vi "Elevator Controller.vi"(8 "error in (no error)":errorcluster, 11 "View Model":T1) -> (0 "error out":errorcluster)   [LabVIEW 2017]
doc: "Handles all elevator operations."
uses:
  View Model/Controls/View Model.ctl
  Configuration/Controls/Config Model.ctl
  Configuration/Controls/Config Data.ctl
  Error Handler/Controls/Error Model.ctl
  Error Handler/Controls/Error Data.ctl
  Error Handler/Controls/Error Type.ctl
  View Model/Controls/Shared Model.ctl
  Controls/Elevator Model.ctl
  Controls/Elevator Location.ctl
  Controls/Elevator CMD Data.ctl
  Controls/Elevator Commands.ctl
  Controls/Elevator Overhead.ctl
  Controls/Elevator States.ctl
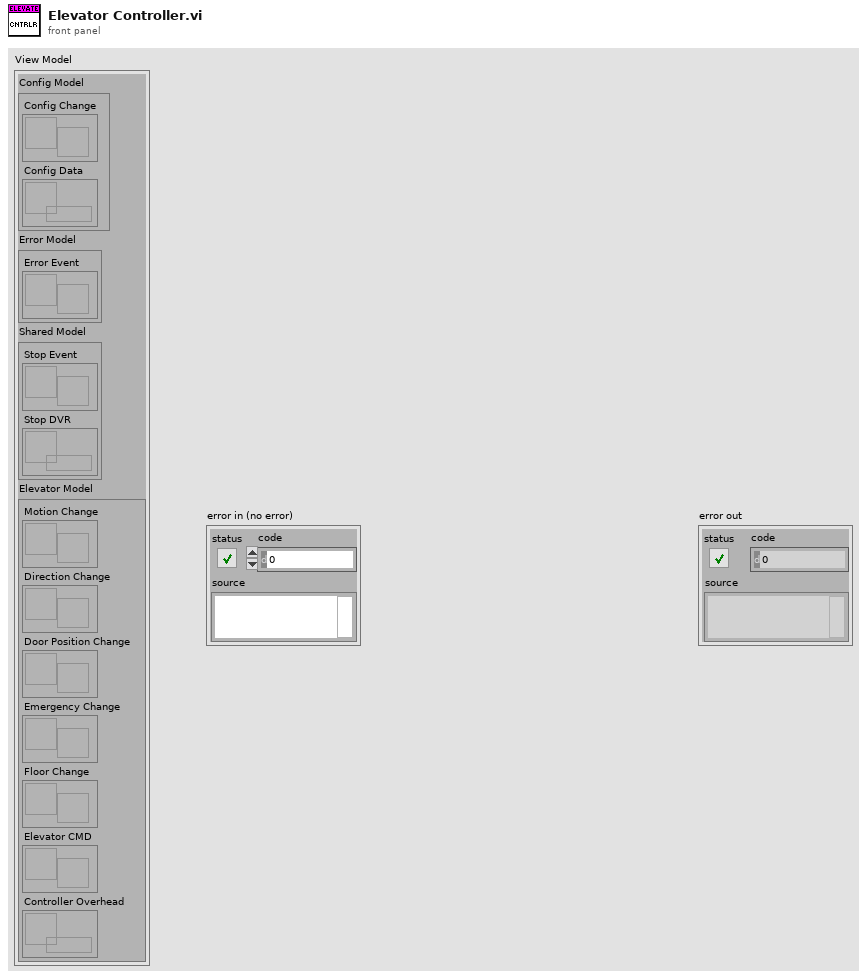
[diagram p1: front panel]
types:
  T1 = typedef "View Model.ctl" = cluster{"Config Model":T2, "Error Model":T3, "Shared Model":T4, "Elevator Model":T5}
  T2 = typedef "Config Model.ctl" = cluster{"Config Change":refnum<user-event>, "Config Data":refnum<data-value>}
  T3 = typedef "Error Model.ctl" = cluster{"Error Event":refnum<user-event>}
  T4 = typedef "Shared Model.ctl" = cluster{"Stop Event":refnum<user-event>, "Stop DVR":refnum<data-value>}
  T5 = typedef "Elevator Model.ctl" = cluster{"Motion Change":refnum<user-event>, "Direction Change":refnum<user-event>, "Door Position Change":refnum<user-event>, "Emergency Change":refnum<user-event>, "Floor Change":refnum<user-event>, "Elevator CMD":refnum<user-event>, "Controller Overhead":refnum<data-value>}
  T6 = typedef "Elevator Commands.ctl" = enum16{"Go Up", "Go Down", "Go to Floor", "Emergency", "Open Doors", "Close Doors"}
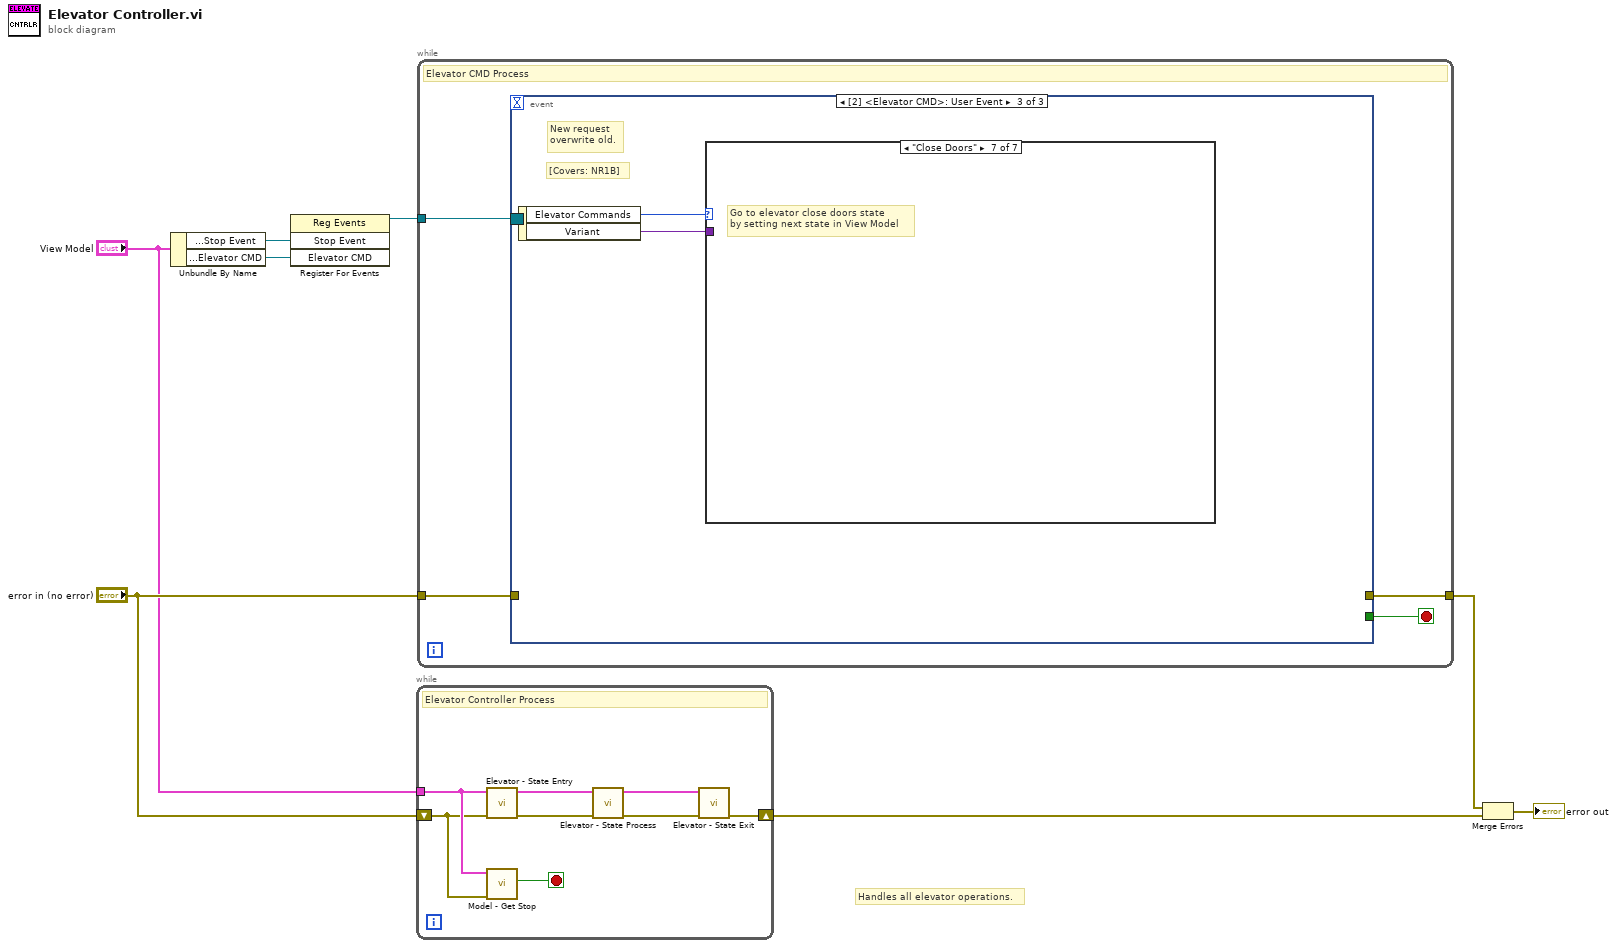
[diagram p0: block diagram]
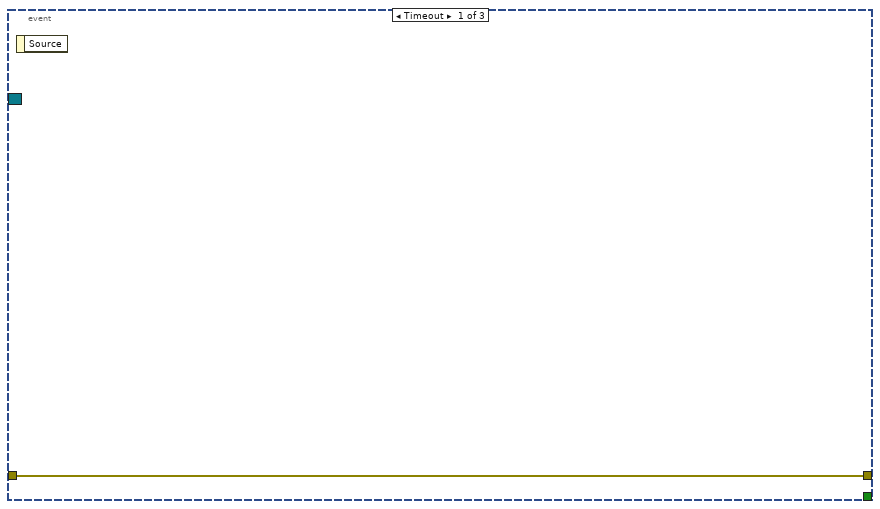
[diagram p2: hidden frame]
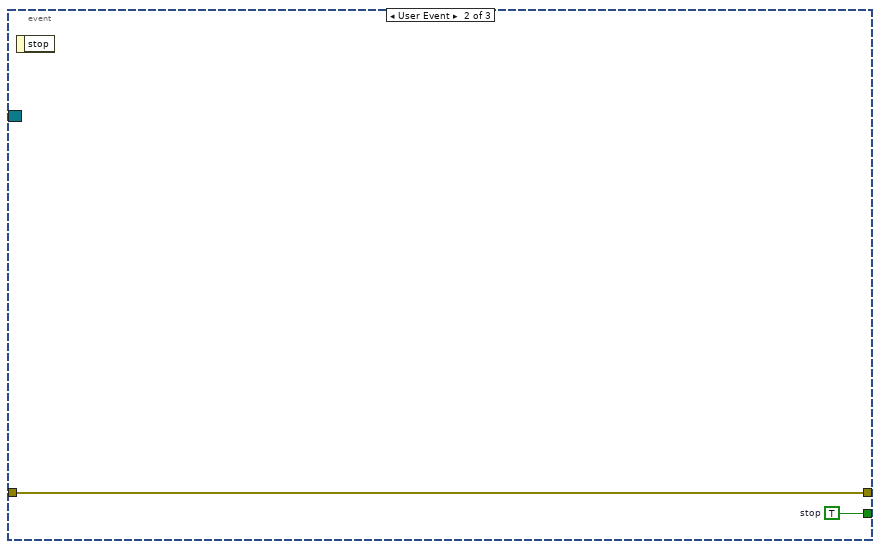
[diagram p3: hidden frame]
diagram:
  # "Handles all elevator operations."
  n1 = Unbundle By Name("View Model") -> ("Shared Model.Stop Event"=w8:refnum<user-event>, "Elevator Model.Elevator CMD"=w7:refnum<user-event>)
  n2 = register-events(w8, w7) -> (reference out=w6:refnum<event-registration>)  [unwired: 2 in, 1 out]
  n3 = while {
    tunnel: "View Model" -> [w12]
    shift-right: [w9] -> w3
    shift-left: "error in (no error)" -> [w11]
    stop <- w10 stop-if-true
    # "Elevator Controller Process"
    n4 = call "Elevator - State Entry.vi"("error in (no error)"=w11, "View Model"=w12) -> ("error out"=w14:errorcluster, "View Model"=w16:T1)  [unwired: 8 in]
    n5 = call "Model - Get Stop.vi"("error in (no error)"=w11, "View Model"=w12) -> ("Stop"=w10:bool)  [unwired: 7 in, 2 out]
    n6 = call "Elevator - State Process.vi"("error in (no error)"=w14, "View Model"=w16) -> ("error out"=w13:errorcluster, "View Model"=w15:T1)  [unwired: 8 in]
    n7 = call "Elevator - State Exit.vi"("error in (no error)"=w13, "View Model"=w15) -> ("error out"=w9:errorcluster)  [unwired: 8 in, 1 out]
  }
  n8 = while {
    tunnel: w6 -> [w20]
    tunnel: "error in (no error)" -> [w19]
    tunnel: [w18] -> w2
    stop <- w17 stop-if-true
    # "Elevator CMD Process"
    n9 = event shown="[2] <Elevator CMD>: User Event" {
      selector: w20 -> [_ _ _]
      dyn-events: _ -> [_ _ _]
      timeout: _ -> [_ _ _]
      tunnel: w19 -> [w21 w22 _]
      tunnel: [w21 w22 _] -> w18
      tunnel: [_ w23 _] -> w17
      event Timeout {
        n10 = event-data() -> ()  [unwired: 1 in, 1 out]
      }
      event User Event {
        w23 = TRUE  # stop
        n11 = event-data() -> ()  [unwired: 1 in, 1 out]
      }
      event User Event {
        # "[Covers: NR1B]"
        # "New request \noverwrite old."
        n12 = event-data() -> ("Elevator Commands"=w25:T6, "Variant"=w24:variant)  [unwired: 1 in]
        n13 = case shown="\"Close Doors\"" w25 {
          tunnel: w24 -> [_ _ _ _ _ _ _]
          frame Default {
          }
          frame "Go Up" {
            # "[Covers: OC3A]"
            # "Go to elevator move up state\nby setting next state in View Model"
          }
          frame "Go Down" {
            # "Go to elevator move down state\nby setting next state in View Model"
          }
          frame "Go to Floor" {
            # "[Covers: WS3]"
            # "[Covers: WS2]"
            # "If on the first floor, set open doors to next state,\nelse set travel state"
            # "Go to elevator move up/down state\nby setting next state in View Model"
          }
          frame "Emergency" {
            # "Go to elevator emergency state\nby setting next state in View Model"
          }
          frame "Open Doors" {
            # "Go to elevator open doors state\nby setting next state in View Model"
          }
          frame "Close Doors" {
            # "Go to elevator close doors state\nby setting next state in View Model"
          }
        }
      }
    }
  }
  n14 = Merge Errors(w2, w3) -> (→"error out":errorcluster)
